vi "script model runner vi.vi"(4 "parameters":T1[](array[typedef]), 6 "indicators":T1[](array[typedef]), 8 "error in":errorcluster, 9 "controls":T1[](array[typedef]), 10 "project directory":path, 11 "VI in":refnum<vi>) -> (0 "error out":errorcluster)   [LabVIEW 2014, in "CD model script.lvlib"]
uses:
  CD model script.lvlib
  interface spec.ctl
  <vilib>/Utility/miscctls.llb/LVPointTypeDef.ctl
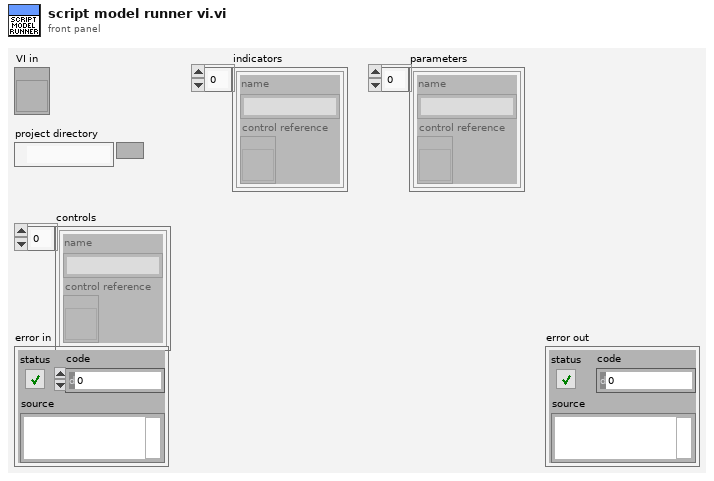
[diagram p1: front panel]
types:
  T1 = typedef "CD model script.lvlib/interface spec.ctl" = cluster{"name":string, "control reference":refnum<vi>}
  T2 = typedef "LVPointTypeDef.ctl" = cluster{"Horizontal":i16, "Vertical":i16}
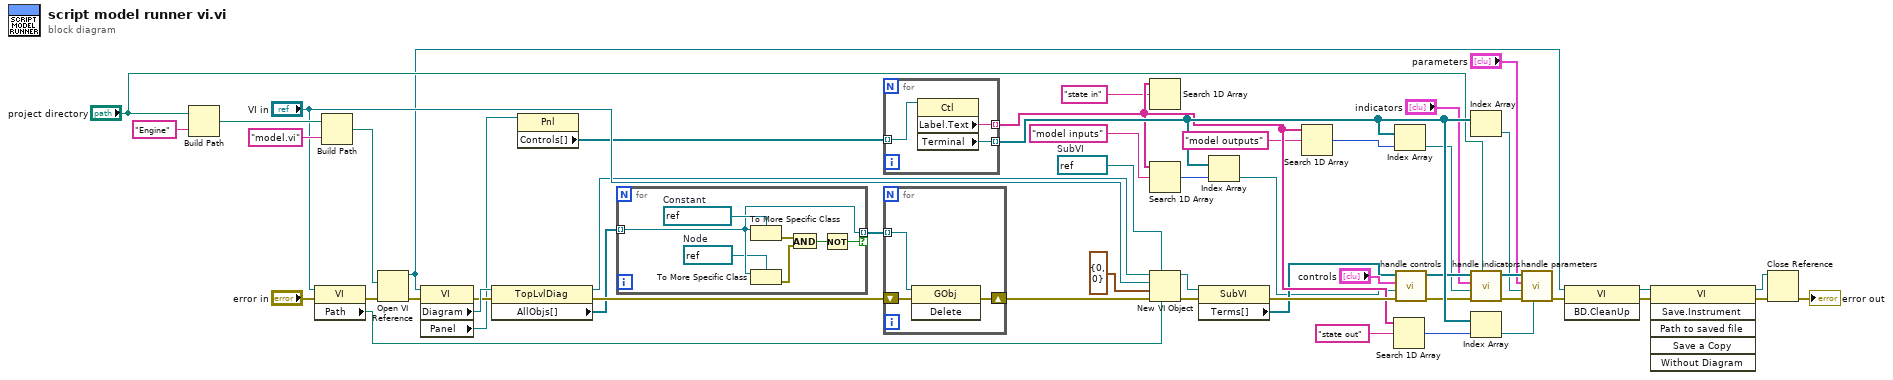
[diagram p0: block diagram]
diagram:
  w40 = refnum<vi> refnum  # SubVI
  n1 = Build Path(base path="project directory", name or relative path="Engine") -> (appended path=w52:path)
  n2 = property class="VI"(reference="VI in", error in="error in") -> (error out=w43:errorcluster, "Path"=w42:path)  [unwired: 1 out]
  n3 = Build Path(base path=w52, name or relative path="model.vi") -> (appended path=w49:path)
  n4 = Open VI Reference(vi path=w49, error in (no error)=w43) -> (vi reference=w4:refnum<vi>, error out=w44:errorcluster)  [unwired: 4 in]
  n5 = property class="VI"(reference=w4, error in=w44) -> (error out=w37:errorcluster, "Diagram"=w38:refnum<vi>, "Panel"=w35:refnum<vi>)  [unwired: 1 out]
  n6 = property class="TopLvlDiag"(reference=w38, error in=w37) -> (reference out=w21:refnum<vi>, error out=w36:errorcluster, "AllObjs[]"=w2:refnum<vi>[])
  n7 = property class="Pnl"(reference=w35) -> ("Controls[]"=w34:refnum<vi>[])  [unwired: 1 in, 2 out]
  n8 = for {
    tunnel: w2 -> [w55] mode=indexing
    tunnel: [w55] -> w1 mode=indexing if=w54
    w53 = refnum<vi> refnum  # Node
    w59 = refnum<vi> refnum  # Constant
    n9 = To More Specific Class(target class=w59, reference=w55) -> (error out=w57:errorcluster)  [unwired: 1 in, 1 out]
    n10 = To More Specific Class(target class=w53, reference=w55) -> (error out=w58:errorcluster)  [unwired: 1 in, 1 out]
    n11 = And(x=w57, y=w58) -> (x .and. y?=w56:bool)
    n12 = Not(x=w56) -> (.not. x?=w54:bool)
  }
  n13 = for {
    tunnel: w34 -> [w62] mode=indexing
    tunnel: [w61] -> w26 mode=indexing
    tunnel: [w60] -> w29 mode=indexing
    n14 = property class="Ctl"(reference=w62) -> ("Label.Text"=w61:string, "Terminal"=w60:refnum<vi>)  [unwired: 1 in, 2 out]
  }
  n15 = for {
    shift-right: [w64] -> w20
    shift-left: w36 -> [w65]
    tunnel: w1 -> [w63] mode=indexing
    n16 = invoke class="GObj" method="Delete"(reference=w63, error in=w65) -> (error out=w64:errorcluster)  [unwired: 1 in, 2 out]
  }
  n17 = Search 1D Array(1D array=w26, element="state in") -> ()  [unwired: 1 in, 1 out]
  n18 = Search 1D Array(1D array=w26, element="model inputs") -> (index of element=w27:i32)  [unwired: 1 in]
  n19 = New VI Object(vi object class=w40, owner refnum=w21, style="VI in", position/next to=T2 {"Horizontal"=0, "Vertical"=0} ("location"), 6:w42, 8:w20) -> (object refnum=w32:refnum<vi>, 0:w33:errorcluster)  [unwired: 2 in]
  n20 = property class="SubVI"(reference=w32, error in=w33) -> (error out=w31:errorcluster, "Terms[]"=w18:refnum<vi>[])  [unwired: 1 out]
  n21 = Index Array(array=w29, index=w27) -> (element=w17:refnum<vi>)
  n22 = Search 1D Array(1D array=w26, element="model outputs") -> (index of element=w30:i32)  [unwired: 1 in]
  n23 = Search 1D Array(1D array=w26, element="state out") -> (index of element=w28:i32)  [unwired: 1 in]
  n24 = Index Array(array=w29, index=w30) -> (element=w13:refnum<vi>)
  n25 = call "handle controls.vi"("error in (no error)"=w31, "ControlTerminal in"=w17, "controls"="controls", "Terms[] in"=w18) -> ("error out"=w16:errorcluster, "Terms[] out"=w15:refnum<vi>[])  [unwired: 6 in]
  n26 = Index Array(array=w29) -> (element=w5:refnum<vi>)  [unwired: 1 in]
  n27 = call "handle indicators.vi"("project directory"="project directory", "error in (no error)"=w16, "ControlTerminal in"=w13, "controls"="indicators", "Terms[] in"=w15) -> ("error out"=w10:errorcluster, "Terms[] out"=w8:refnum<vi>[])  [unwired: 5 in]
  n28 = Index Array(array=w29, index=w28) -> (element=w6:refnum<vi>)
  n29 = call "handle parameters.vi"("state out"=w6, "error in (no error)"=w10, "state in"=w5, "controls"="parameters", "Terms[] in"=w8) -> ("error out"=w9:errorcluster)  [unwired: 5 in, 1 out]
  n30 = invoke class="VI" method="BD.CleanUp"(reference=w4, error in=w9) -> (reference out=w3:refnum<vi>, error out=w11:errorcluster)  [unwired: 1 in, 1 out]
  n31 = invoke class="VI" method="Save.Instrument"(reference=w3, error in=w11) -> (reference out=w47:refnum<vi>, error out=w48:errorcluster)  [unwired: 4 in, 4 out]
  n32 = Close Reference(reference=w47, error in (no error)=w48) -> (error out=→"error out":errorcluster)
